vi "setpoints.vi"() -> ()   [LabVIEW 2013]
uses:
  <vilib>/Utility/file.llb/Read From Spreadsheet File (DBL).vi
  Robot Global Data.vi
panel:
  in  "Default File":i32
  out "Number of Auton Files":i64
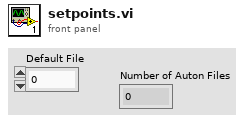
[diagram p1: front panel]
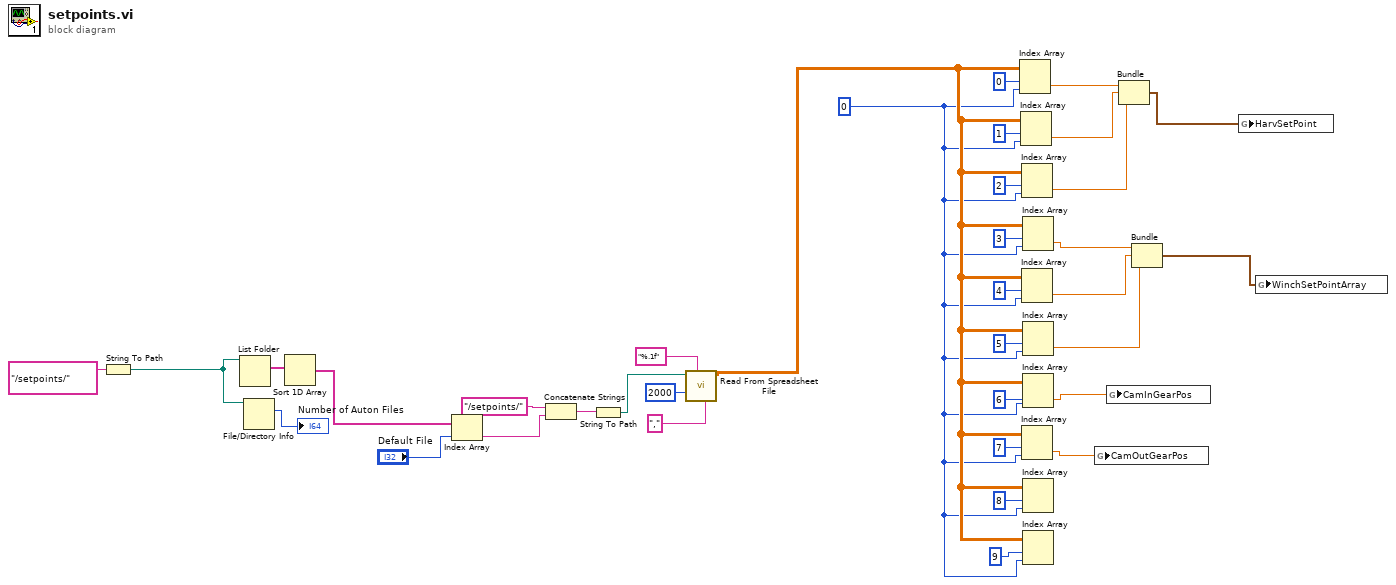
[diagram p0: block diagram]
diagram:
  w11 = 0
  n1 = String To Path(string="/setpoints/") -> (path=w26:path)
  n2 = List Folder(path=w26) -> (filenames=w27:string[])  [unwired: 1 in, 5 out]
  n3 = File/Directory Info(path=w26) -> (size=→"Number of Auton Files":i64)  [unwired: 1 in, 6 out]
  n4 = Sort 1D Array(array=w27) -> (sorted array=w29:string[])
  n5 = Index Array(array=w29, index="Default File") -> (element=w24:string)
  n6 = Concatenate Strings("/setpoints/" ("string"), w24) -> (w32:string)
  n7 = String To Path(string=w32) -> (path=w31:path)
  n8 = call-poly <vilib>:"Read From Spreadsheet File.vi"("delimiter (\\t)"="," ("delimiter (\\t)"), "format (%.3f)"="%.1f", "number of rows (all:-1)"=2000, "file path (dialog if empty)"=w31) -> ("all rows"=w12:dbl[][])  [unwired: 1 in, 6 out]
  n9 = Index Array(array=w12, index (row)=0, index (col)=w11) -> (element=w10:dbl)
  n10 = Index Array(array=w12, index (row)=1, index (col)=w11) -> (element=w9:dbl)
  n11 = Index Array(array=w12, index (row)=2, index (col)=w11) -> (element=w8:dbl)
  n12 = Index Array(array=w12, index (row)=4, index (col)=w11) -> (element=w5:dbl)
  n13 = Index Array(array=w12, index (row)=7, index (col)=w11) -> (element=w2:dbl)
  n14 = Index Array(array=w12, index (row)=3, index (col)=w11) -> (element=w6:dbl)
  n15 = Index Array(array=w12, index (row)=5, index (col)=w11) -> (element=w4:dbl)
  n16 = Index Array(array=w12, index (row)=6, index (col)=w11) -> (element=w1:dbl)
  n17 = Index Array(array=w12, index (row)=8, index (col)=w11) -> ()  [unwired: 1 out]
  n18 = Index Array(array=w12, index (row)=9, index (col)=w11) -> ()  [unwired: 1 out]
  n19 = global write "Robot Global Data.vi" "CamOutGearPos"(w2) -> ()
  n20 = global write "Robot Global Data.vi" "CamInGearPos"(w1) -> ()
  n21 = Bundle(w10, w9, w8) -> (w7:cluster{dbl, dbl, dbl})  [unwired: 1 in]
  n22 = Bundle(w6, w5, w4) -> (w3:cluster{dbl, dbl, dbl})  [unwired: 1 in]
  n23 = global write "Robot Global Data.vi" "HarvSetPoint"(w7) -> ()
  n24 = global write "Robot Global Data.vi" "WinchSetPointArray"(w3) -> ()
